vi "Instrument Name and Icon UI.vi"(11 "Template Name":string="Framework-Template") -> ()   [LabVIEW 2019, in "ProjectItem.lvclass"]
uses:
  ProjectItem.lvclass
  Typedefs/ClassData--Cluster.ctl
  <vilib>/LabVIEW Icon API/lv_icon/Classes/Icon/Icon.lvclass
  <vilib>/LabVIEW Icon API/LabVIEW Icon API.lvlib
panel:
  in  "Launch Icon Editor":bool
  in  "Cancel":bool
  out "Instrument UI Library Icon":picture
  out "Instrument Library Icon":picture
  in  "OK":bool
  in  "Icon Text":string="NEW"
  in  "New Name":string="NewInstrument"
  in  "Instrument UI Color":u32(colorbox)=12123647
  in  "Instrument UI Text Color":u32(colorbox)
  in  "Instrument Color":u32(colorbox)=6618880
  in  "Instrument Text Color":u32(colorbox)
  # "1. Rename your new project and classes"
  # "2. Design a new icon"
  # "3. Write out"
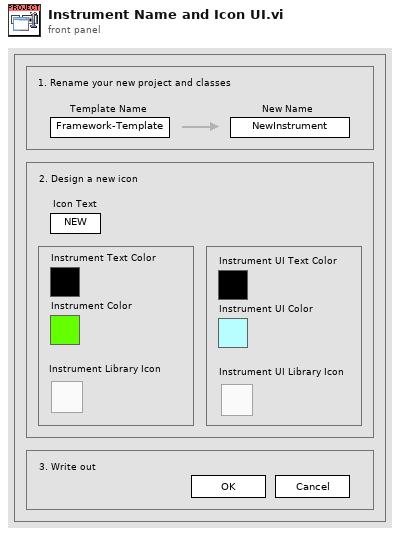
[diagram p1: front panel]
types:
  T1 = enum32{"Invalid", "Standard", "Closed", "Hidden", "Minimized", "Maximized"}
  T2 = enum32{"invalid app kind", "Development System", "Run Time System", "Student Edition", "Embedded LabVIEW", "Evaluation", "Custom"}
  T3 = typedef "ProjectItem.lvclass/ClassData--Cluster.ctl" = cluster{"Name":string, "Icon Text":string, "Text Color":u32, "Color":u32, "Icon":refnum<class "Icon.lvclass">}
  T4 = cluster{"Core":cluster{"Current VI Reference":refnum<vi>, "Close Panel on Exit?":bool}, "Replace Template":string, "Instrument":T3, "Instrument UI":T3, "ProjectItem":refnum<class "ProjectItem.lvclass">}
  T5 = cluster{"Current VI Reference":refnum<vi>, "Close Panel on Exit?":bool}
  T6 = typedef "imagedata.ctl" = cluster{"image type":i32, "image depth":i32, "image":u8[], "mask":u8[], "colors":u32[], "Rectangle":cluster{"left":i16, "top":i16, "right":i16, "bottom":i16}}
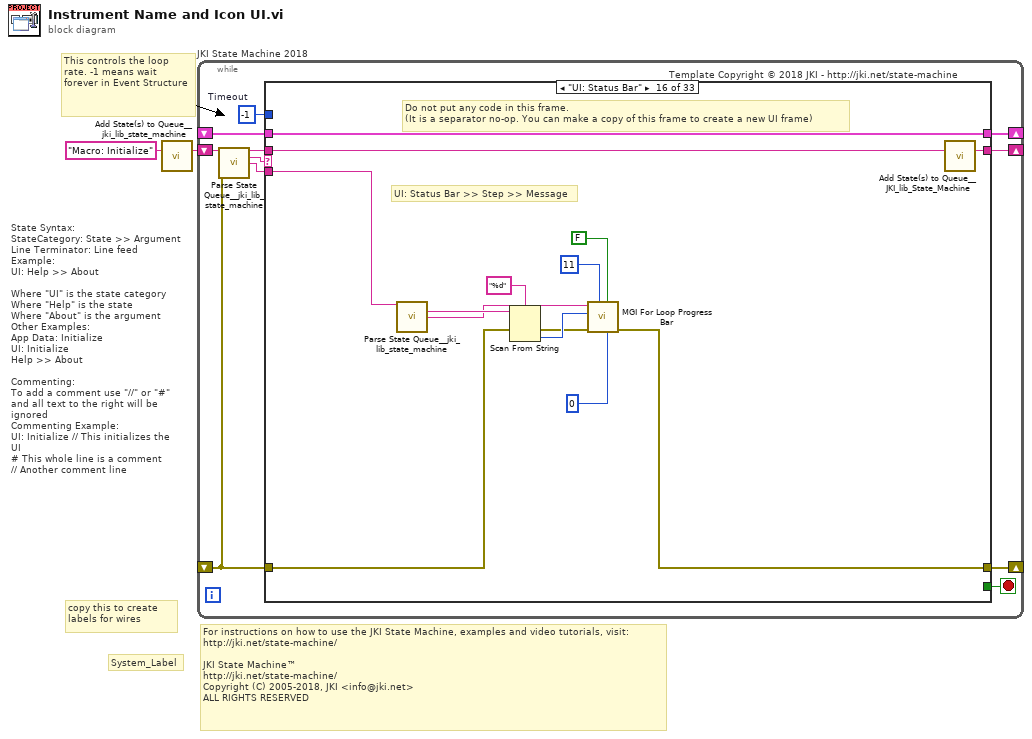
[diagram p0: block diagram]
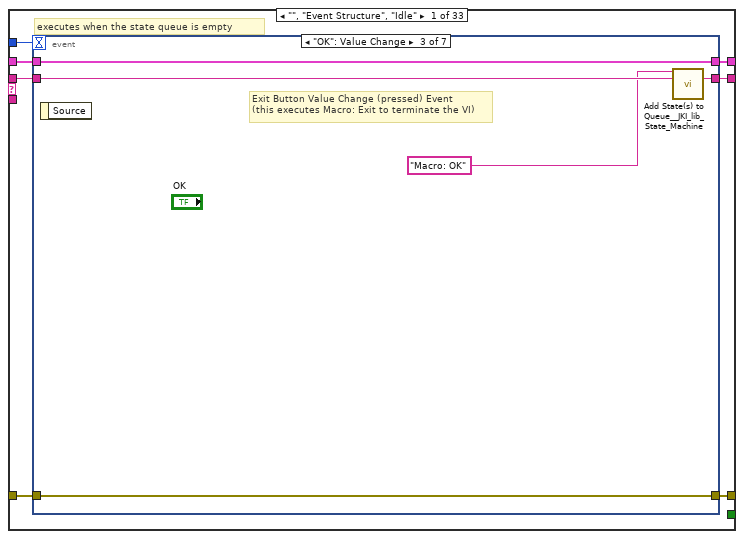
[diagram p2: hidden frame]
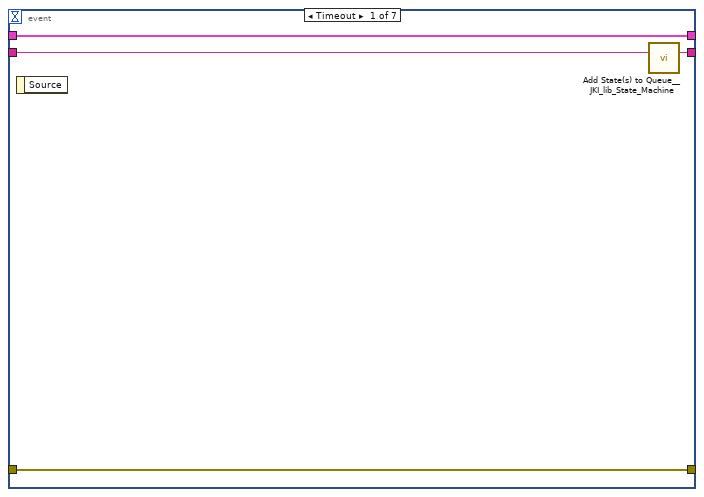
[diagram p3: hidden frame]
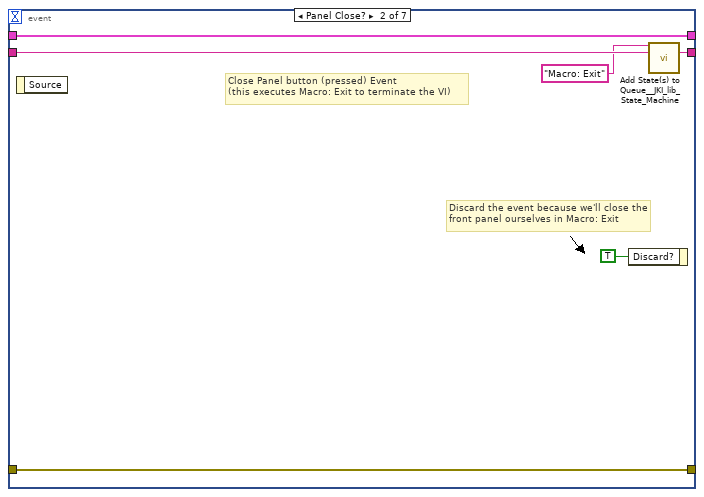
[diagram p4: hidden frame]
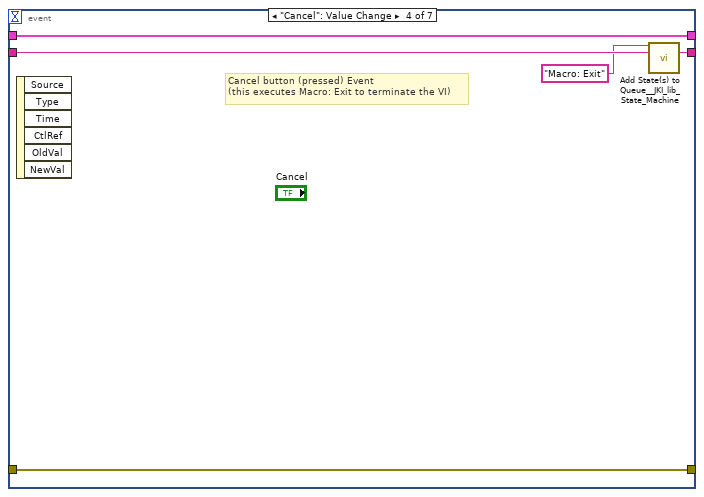
[diagram p5: hidden frame]
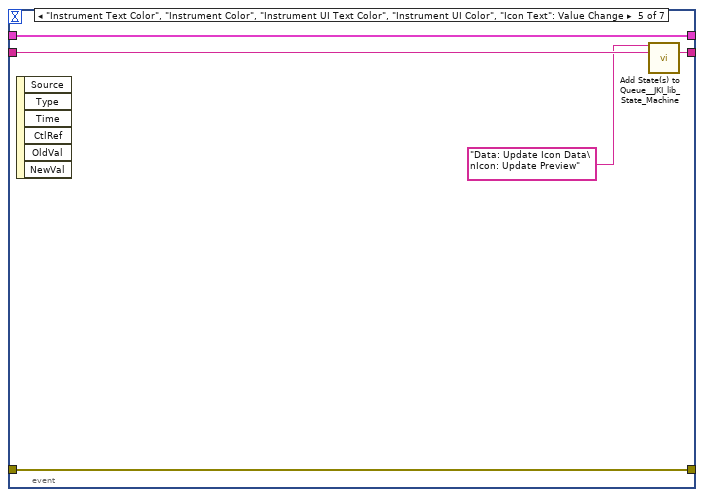
[diagram p6: hidden frame]
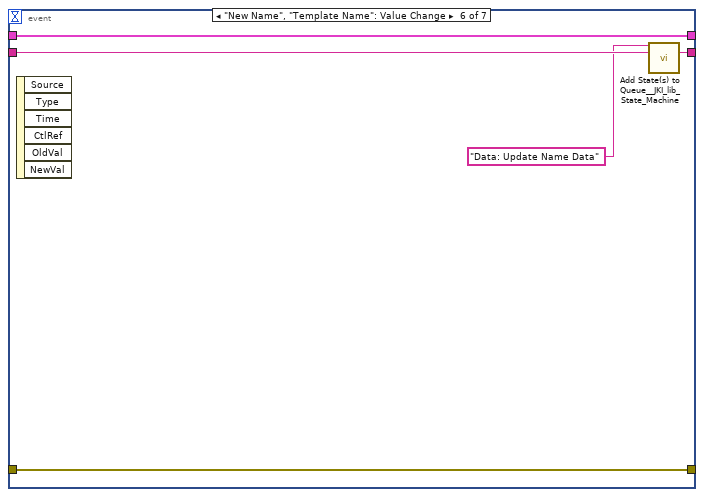
[diagram p7: hidden frame]
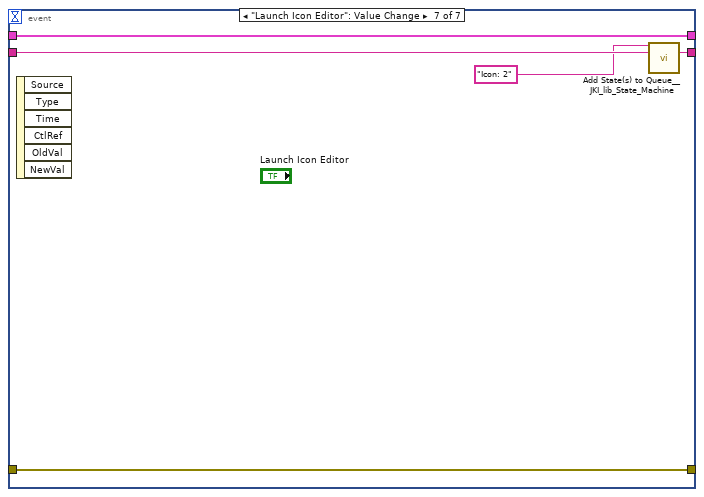
[diagram p8: hidden frame]
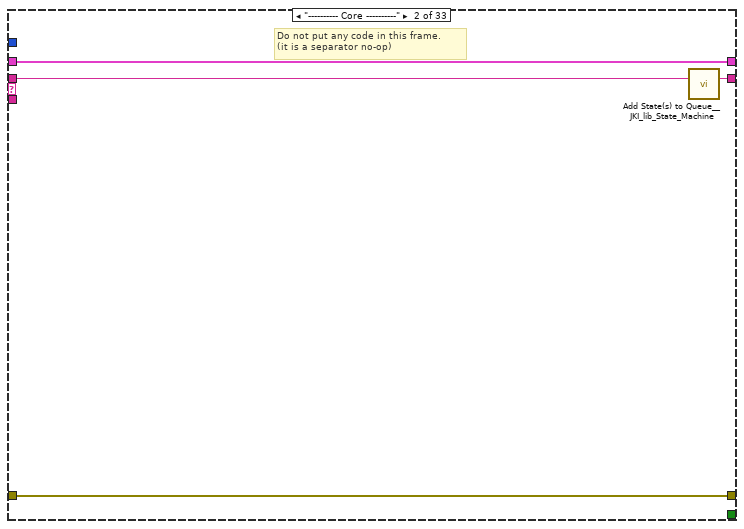
[diagram p9: hidden frame]
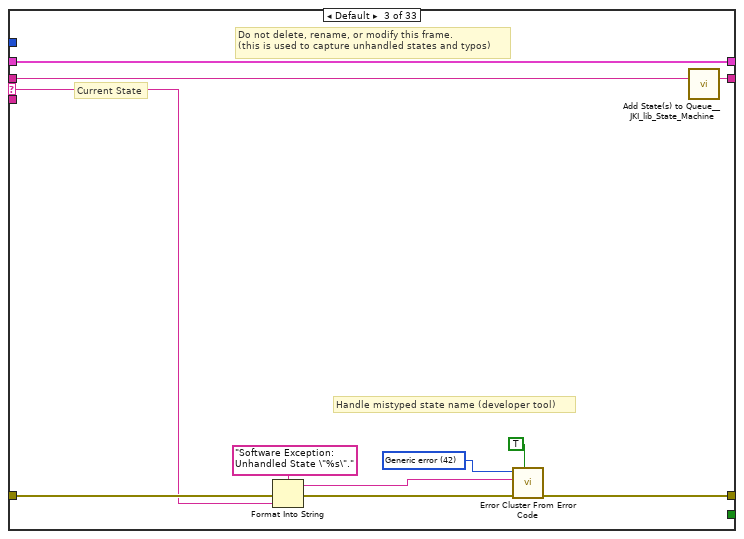
[diagram p10: hidden frame]
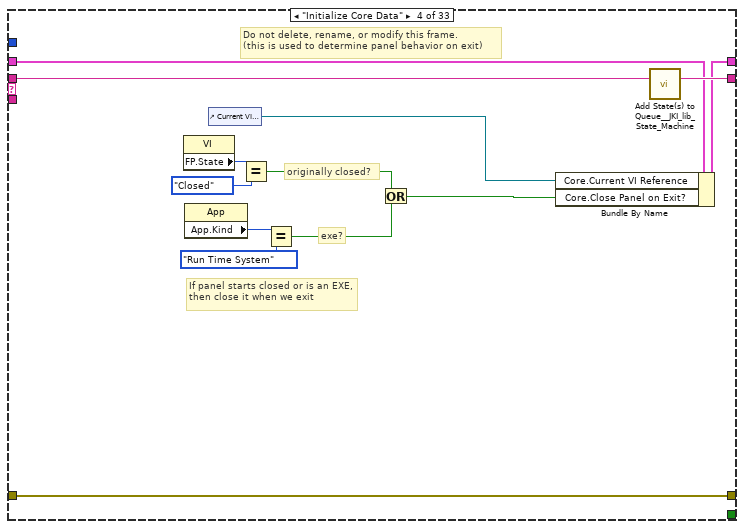
[diagram p11: hidden frame]
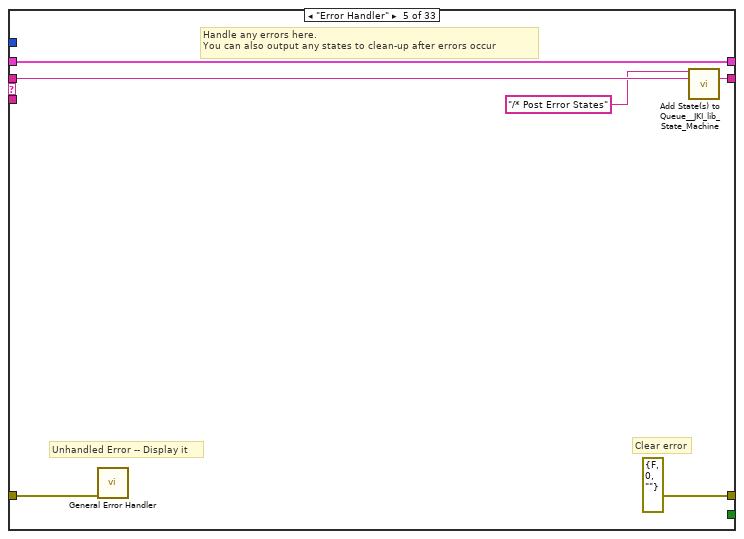
[diagram p12: hidden frame]
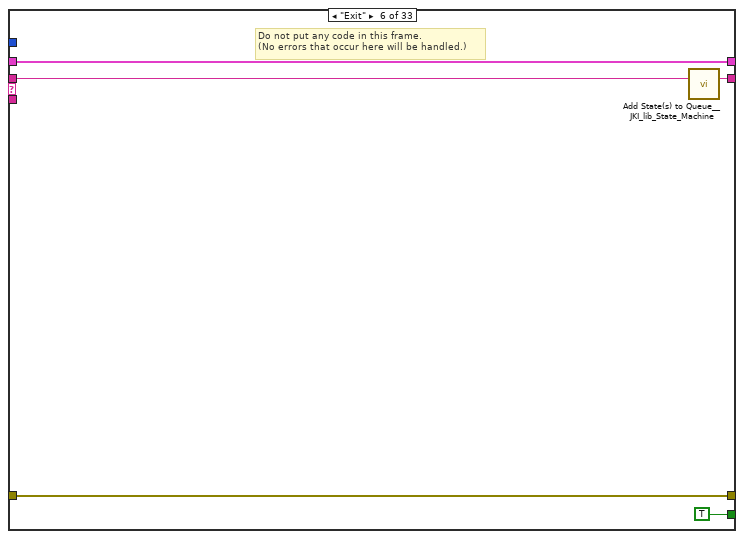
[diagram p13: hidden frame]
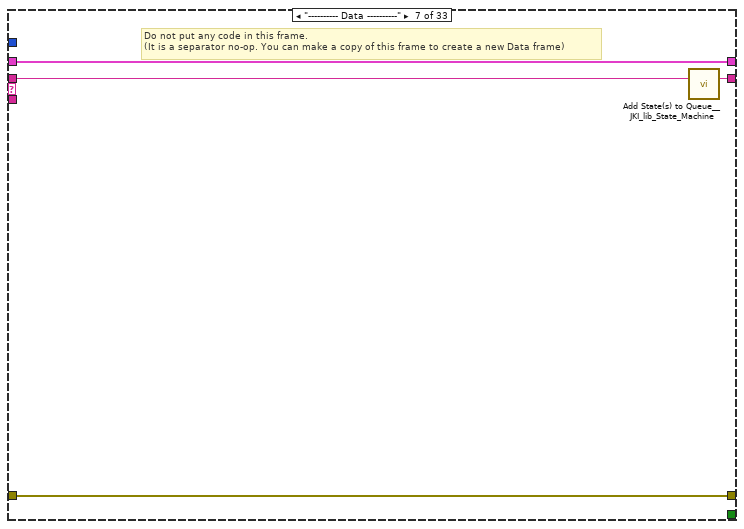
[diagram p14: hidden frame]
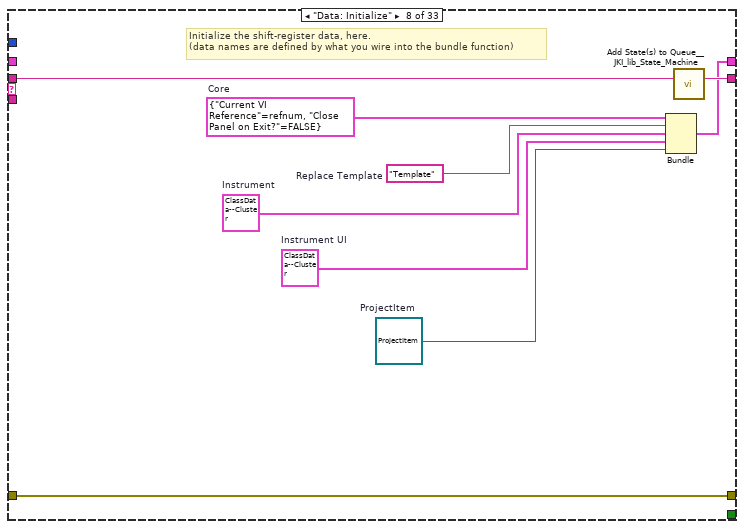
[diagram p15: hidden frame]
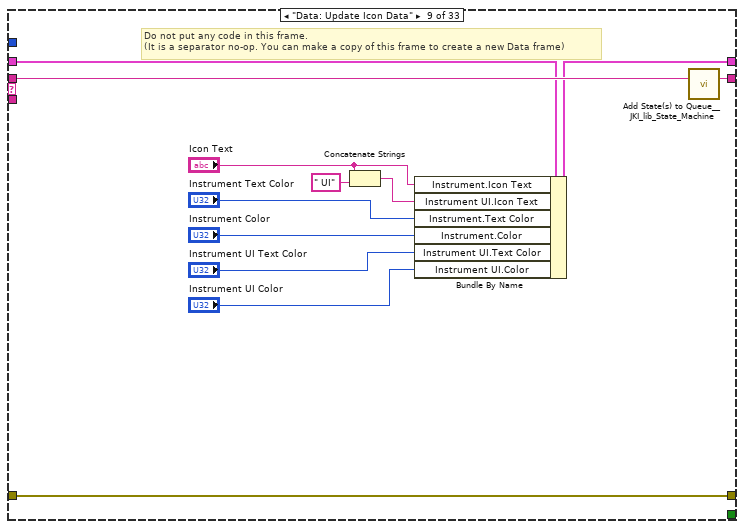
[diagram p16: hidden frame]
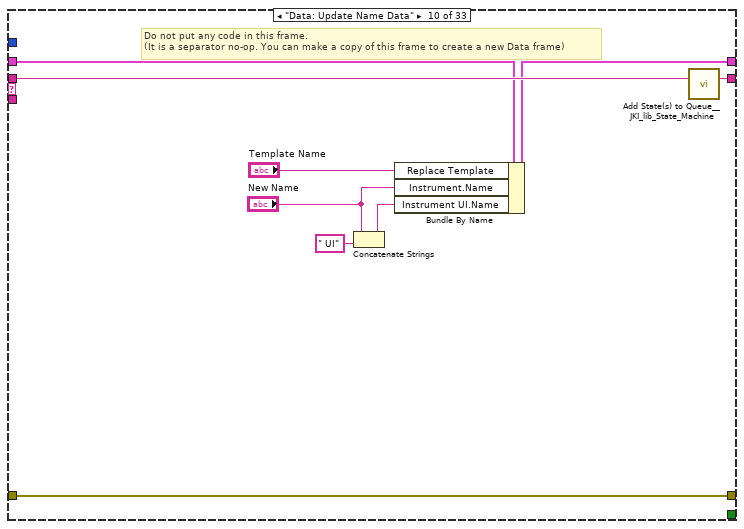
[diagram p17: hidden frame]
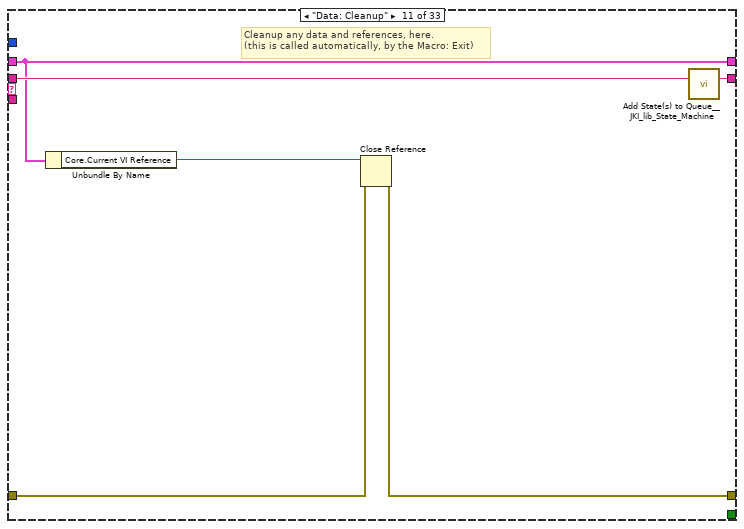
[diagram p18: hidden frame]
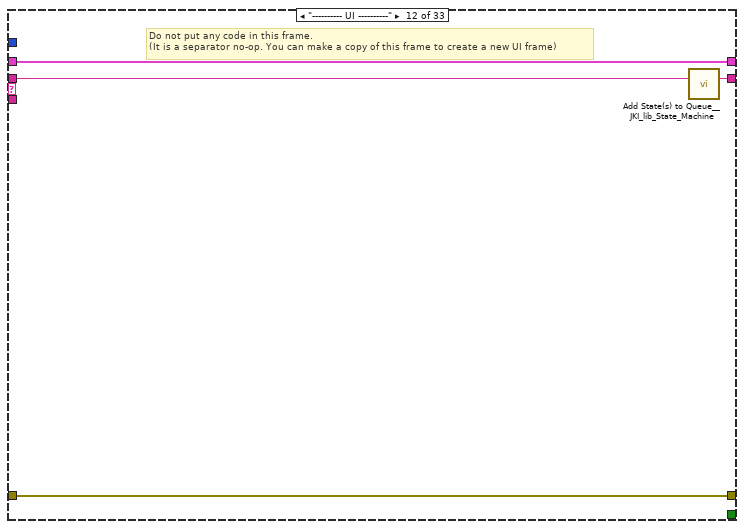
[diagram p19: hidden frame]
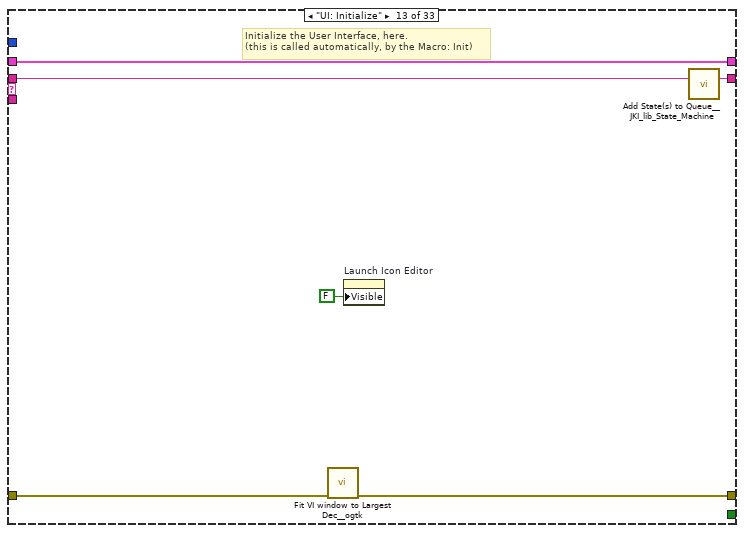
[diagram p20: hidden frame]
diagram:
  # "For instructions on how to use the JKI State Machine, examples and video tutorials, visit:\nhttp://jki.net/state-machine/\n\nJKI State Machine™\nhttp://jki.net/state-machine/\nCopyright (C) 2005-2018, JKI <info@jki.net>\nALL RIGHTS RESERVED"
  # "State Syntax:\nStateCategory: State >> Argument\nLine Terminator: Line feed\nExample:\nUI: Help >> About\n\nWhere \"UI\" is the state category\nWhere \"Help\" is the state\nWhere \"About\" is the argument\nOther Examples:\nApp Data: Initialize\nUI: Initialize\nHelp >> About\n\nCommenting:\nTo add a comment use \"//\" or \"#\" and all text to the right will be ignored\nCommenting Example:\nUI: Initialize // This initializes the UI\n# This whole line is a comment\n// Another comment line"
  # "copy this to create labels for wires"
  # "This controls the loop rate. -1 means wait forever in Event Structure"
  # "System_Label"
  n1 = call <vilib>:"Add State(s) to Queue__jki_lib_state_machine.vi"("State(s) in (\"\")"="Macro: Initialize") -> ("States Out"=w2:string)  [unwired: 14 in]
  n2 = while "JKI State Machine 2018" {
    shift-right: [w6] -> _
    shift-left: _ -> [w5]
    shift-right: [w9] -> _
    shift-left: _ -> [w3]
    shift-right: [w8] -> _
    shift-left: w2 -> [w10]
    stop <- w7 stop-if-true
    w4 = -1  # Timeout
    # "Template Copyright © 2018 JKI - http://jki.net/state-machine"
    n3 = call <vilib>:"Parse State Queue__jki_lib_state_machine.vi"("State Queue"=w10, "Error In (no error)"=w3) -> ("Remaining States"=w12:string, "Current State"=w13:string, "Arguments"=w11:string)  [unwired: 11 in]
    n4 = case shown="\"UI: Status Bar\"" w13 {
      selector: w13 -> [_ _ w60 _ _ _ _ _ _ _ _ _ _ _ _ _ _ _ _ _ _ _ _ _ _ _ _ _ _ _ _ _ _]
      tunnel: w12 -> [w20 w59 w64 w83 w89 w94 w98 w107 w119 w128 w134 w138 w144 w150 w161 w240 w244 w249 w265 w281 w285 w305 w320 w324 w334 w342 w350 w358 w366 w374 w384 w394 w400]
      tunnel: w11 -> [_ _ _ _ _ _ _ _ _ _ _ _ _ w145 w155 w237 _ _ _ _ _ _ _ _ _ _ _ _ _ _ _ _ _]
      tunnel: w5 -> [w18 w56 w62 w76 w86 w92 w95 _ w114 w125 w130 w135 w142 w148 w157 w238 w241 w246 w262 w278 w282 w296 w310 w321 w330 w339 w347 w355 w363 w371 w379 w389 w398]
      tunnel: [w17 w57 w66 w80 errorcluster {"status"=FALSE, "code"=0, "source"=""} ("error out") w91 w96 w104 w117 w126 w131 w136 w141 w146 w158 w228 w242 w247 w263 w279 w283 w299 w312 w322 w327 w336 w344 w351 w359 w367 w381 w391 w395] -> w9
      tunnel: w3 -> [w16 w57 w65 w80 w85 w91 w96 w104 w117 w126 w129 w136 w140 w147 w159 w229 w242 w247 w263 w279 w283 w301 w317 w322 w326 w335 w343 w352 w360 w368 w382 w392 w396]
      tunnel: [w19 w58 w63 w82 w88 w93 w97 w106 w118 w127 w133 w137 w143 w149 w160 w239 w243 w248 w264 w280 w284 w304 w319 w323 w333 w341 w349 w357 w365 w373 w383 w393 w399] -> w8
      tunnel: [_ _ _ _ _ TRUE _ _ _ _ _ _ _ _ _ _ _ _ _ _ _ _ _ _ _ _ _ _ _ _ _ _ _] -> w7
      tunnel: [w15 w56 w62 w81 w86 w92 w95 w105 w113 w124 w130 w135 w142 w148 w157 w238 w241 w246 w262 w278 w282 w297 w316 w321 w329 w338 w346 w354 w362 w370 w380 w390 w398] -> w6
      tunnel: w4 -> [w14 _ _ _ _ _ _ _ _ _ _ _ _ _ _ _ _ _ _ _ _ _ _ _ _ _ _ _ _ _ _ _ _]
      frame "", "Event Structure", "Idle" {
        # "executes when the state queue is empty"
        n5 = event shown="[2] \"OK\": Value Change" {
          selector: _ -> [_ _ _ _ _ _ _]
          dyn-events: _ -> [_ _ _ _ _ _ _]
          timeout: w14 -> [_ _ _ _ _ _ _]
          tunnel: w20 -> [w24 w30 w35 w40 w45 w50 w55]
          tunnel: [w23 w29 w34 w39 w44 w49 w54] -> w19
          tunnel: w18 -> [w21 w27 w32 w37 w41 w46 w51]
          tunnel: [w22 w28 w33 w38 w43 w48 w53] -> w17
          tunnel: w16 -> [w22 w28 w33 w38 w43 w48 w53]
          tunnel: [w21 w27 w32 w37 w41 w46 w51] -> w15
          event Timeout {
            n6 = event-data() -> ()  [unwired: 1 in, 1 out]
            n7 = call <vilib>:"Add State(s) to Queue__JKI_lib_State_Machine.vi"("State(s) in (\"\")"=w24) -> ("States Out"=w23:string)  [unwired: 14 in]
          }
          event Panel Close? {
            # "Discard the event because we'll close the front panel ourselves in Macro: Exit"
            # "Close Panel button (pressed) Event\n(this executes Macro: Exit to terminate the VI)"
            n8 = event-data() -> ()  [unwired: 1 in, 1 out]
            n9 = event-data("Discard?"=TRUE) -> ()  [unwired: 1 in, 1 out]
            n10 = call <vilib>:"Add State(s) to Queue__JKI_lib_State_Machine.vi"("State(s) in Front (\"\")"="Macro: Exit", "State(s) in (\"\")"=w30) -> ("States Out"=w29:string)  [unwired: 13 in]
          }
          event "OK": Value Change {
            # "Exit Button Value Change (pressed) Event\n(this executes Macro: Exit to terminate the VI)"
            n11 = event-data() -> ()  [unwired: 1 in, 1 out]
            n12 = call <vilib>:"Add State(s) to Queue__JKI_lib_State_Machine.vi"("State(s) in Front (\"\")"="Macro: OK", "State(s) in (\"\")"=w35) -> ("States Out"=w34:string)  [unwired: 13 in]
          }
          event "Cancel": Value Change {
            # "Cancel button (pressed) Event\n(this executes Macro: Exit to terminate the VI)"
            n13 = event-data() -> ()  [unwired: 1 in, 6 out]
            n14 = call <vilib>:"Add State(s) to Queue__JKI_lib_State_Machine.vi"("State(s) in Front (\"\")"="Macro: Exit", "State(s) in (\"\")"=w40) -> ("States Out"=w39:string)  [unwired: 13 in]
          }
          event "Instrument Text Color", "Instrument Color", "Instrument UI Text Color", "Instrument UI Color", "Icon Text": Value Change {
            n15 = event-data() -> ()  [unwired: 1 in, 6 out]
            n16 = call <vilib>:"Add State(s) to Queue__JKI_lib_State_Machine.vi"("State(s) in Front (\"\")"="Data: Update Icon Data\nIcon: Update Preview", "State(s) in (\"\")"=w45) -> ("States Out"=w44:string)  [unwired: 13 in]
          }
          event "New Name", "Template Name": Value Change {
            n17 = event-data() -> ()  [unwired: 1 in, 6 out]
            n18 = call <vilib>:"Add State(s) to Queue__JKI_lib_State_Machine.vi"("State(s) in Front (\"\")"="Data: Update Name Data", "State(s) in (\"\")"=w50) -> ("States Out"=w49:string)  [unwired: 13 in]
          }
          event "Launch Icon Editor": Value Change {
            n19 = event-data() -> ()  [unwired: 1 in, 6 out]
            n20 = call <vilib>:"Add State(s) to Queue__JKI_lib_State_Machine.vi"("State(s) in Front (\"\")"="Icon: 2", "State(s) in (\"\")"=w55) -> ("States Out"=w54:string)  [unwired: 13 in]
          }
        }
      }
      frame "---------- Core ----------" {
        # "Do not put any code in this frame.\n(it is a separator no-op)"
        n21 = call <vilib>:"Add State(s) to Queue__JKI_lib_State_Machine.vi"("State(s) in (\"\")"=w59) -> ("States Out"=w58:string)  [unwired: 14 in]
      }
      frame Default {
        w69 = 42 items=["No error", "Argument error", "Memory is full", "Out of zone", "End of file", "File already open", "Generic file I/O error", "File not found", "File permission error", "Disk is full", "Duplicate path", "Too many files open", "System feature not enabled", "Resource file not found", "Cannot add resource", "Resource not found", "Image not found", "Image memory error", "Pen does not exist", "Config type invalid", "Config token not found", "Config parse error", "Config memory error", "Bad external code format", "Bad external code offset", "External code not present", "Null window", "Destroy window error", "Null menu", "Print aborted", "Bad print record", "Print driver error", "Windows error during printing", "Memory error during printing", "Print dialog error", "Generic print error", "Invalid device refnum", "Device not found", "Device parameter error", "Device unit error", "Cannot open device", "Device call aborted", "Generic error", "Cancelled by user", "Object ID too low", "Object ID too high", "Object not in heap", "Unknown heap", "Unknown object (invalid DefProc)", "Unknown object (DefProc not in table)", "Message out of range", "Invalid (null) method", "Unknown message", "Manager call not supported", "Bad address", "Network operation in progress", "Network operation timed out", "Connection is busy", "Network attribute not supported", "Network error", "Address in use", "System out of memory", "Connection aborted", "Connection refused", "Not connected", "Already connected", "Connection closed", "Initialization error (interapplication manager)", "Bad occurrence", "Wait on unbound occurrence handler", "Occurrence queue overflow", "Datalog type conflict", "Unused", "Unrecognized type (interapplication manager)", "Memory corrupt", "Failed to make temporary DLL", "Old CIN version", "Drag socket not found", "Failed to load drop-object", "Failed to register OLE object", "Failed to release OLE object", "Format specifier type mismatch", "Unknown format specifier", "Too few format specifiers", "Too many format specifiers", "Scan failed", "Newer CIN version", "Error converting to variant", "Runtime menu error", "Password tampered", "Variant attribute not found", "Incompatible variant data type", "Event data is not available", "Event Store is not present", "Occurrence is not found", "Event Queue is not created", "Event info is not available", "Refnum passed is NULL", "Error retrieving Class GUID", "Error retrieving CoClass GUID", "Error retrieving TypeLib GUID.", "Bad built application magic bytes.", "Specific driver is different from the specific driver associated with the Logical Name.", "There is no session opened to the class driver.", "Max Error", "MAX - Error with config objects", "MAX - Error loading configuration", "MAX - Group not supported"]
        # "Current State"
        # "Do not delete, rename, or modify this frame.\n(this is used to capture unhandled states and typos)"
        # "Handle mistyped state name (developer tool)"
        n22 = Format Into String(format string="Software Exception: Unhandled State \"%s\"." ("message"), error in=w65, w60) -> (resulting string=w68:string, error out=w67:errorcluster)  [unwired: 1 in]
        n23 = call <vilib>:"Error Cluster From Error Code.vi"("show call chain? (False)"=TRUE, "error in (no error)"=w67, "error message (\"\")"=w68, "error code (0)"=w69) -> ("error out"=w66:errorcluster)  [unwired: 5 in]
        n24 = call <vilib>:"Add State(s) to Queue__JKI_lib_State_Machine.vi"("State(s) in (\"\")"=w64) -> ("States Out"=w63:string)  [unwired: 14 in]
      }
      frame "Initialize Core Data" {
        # "Do not delete, rename, or modify this frame.\n(this is used to determine panel behavior on exit)"
        # "originally closed?"
        # "exe?"
        # "If panel starts closed or is an EXE, then close it when we exit"
        n25 = property class="VI"() -> ("FP.State"=w73:T1)  [unwired: 2 in, 2 out]
        n26 = property class="App"() -> ("App.Kind"=w79:T2)  [unwired: 2 in, 2 out]
        n27 = control-ref of="Current VI Reference"() -> (w74:refnum<vi>)
        n28 = Equal?(x=w73, y=T1."Closed" ("Front Panel Window:State")) -> (x = y?=w71:bool)
        n29 = Equal?(x=w79, y=T2."Run Time System" ("Application:Kind")) -> (x = y?=w77:bool)
        n30 = Or(x=w71, y=w77) -> (x .or. y?=w75:bool)
        n31 = Bundle By Name(cluster=w76, "Core.Current VI Reference"=w74, "Core.Close Panel on Exit?"=w75) -> (w81:T4)
        n32 = call <vilib>:"Add State(s) to Queue__JKI_lib_State_Machine.vi"("State(s) in (\"\")"=w83) -> ("States Out"=w82:string)  [unwired: 14 in]
      }
      frame "Error Handler" {
        # "Unhandled Error -- Display it"
        # "Handle any errors here.\nYou can also output any states to clean-up after errors occur"
        # "Clear error"
        n33 = call <vilib>:"General Error Handler.vi"("error in (no error)"=w85) -> ()  [unwired: 10 in, 5 out]
        n34 = call <vilib>:"Add State(s) to Queue__JKI_lib_State_Machine.vi"("State(s) in Front (\"\")"="/* Post Error States", "State(s) in (\"\")"=w89) -> ("States Out"=w88:string)  [unwired: 13 in]
      }
      frame "Exit" {
        # "Do not put any code in this frame.\n(No errors that occur here will be handled.)"
        n35 = call <vilib>:"Add State(s) to Queue__JKI_lib_State_Machine.vi"("State(s) in (\"\")"=w94) -> ("States Out"=w93:string)  [unwired: 14 in]
      }
      frame "---------- Data ----------" {
        # "Do not put any code in this frame.\n(It is a separator no-op. You can make a copy of this frame to create a new Data frame)"
        n36 = call <vilib>:"Add State(s) to Queue__JKI_lib_State_Machine.vi"("State(s) in (\"\")"=w98) -> ("States Out"=w97:string)  [unwired: 14 in]
      }
      frame "Data: Initialize" {
        w99 = T3 {"Name"="NewInstrument", "Icon Text"="NewInstrument", "Text Color"=6618880, "Color"=6618880, "Icon"=refnum}  # Instrument UI
        w101 = refnum<class "ProjectItem.lvclass"> refnum  # ProjectItem
        w102 = T3 {"Name"="NewInstrument", "Icon Text"="NewInstrument", "Text Color"=6618880, "Color"=6618880, "Icon"=refnum}  # Instrument
        w100 = "Template"  # Replace Template
        w103 = T5 {"Current VI Reference"=refnum, "Close Panel on Exit?"=FALSE}  # Core
        # "Initialize the shift-register data, here.\n(data names are defined by what you wire into the bundle function)"
        n37 = Bundle("Core"=w103, "Replace Template"=w100, "Instrument"=w102, "Instrument UI"=w99, "ProjectItem"=w101) -> (w105:T4)  [unwired: 1 in]
        n38 = call <vilib>:"Add State(s) to Queue__JKI_lib_State_Machine.vi"("State(s) in (\"\")"=w107) -> ("States Out"=w106:string)  [unwired: 14 in]
      }
      frame "Data: Update Icon Data" {
        # "Do not put any code in this frame.\n(It is a separator no-op. You can make a copy of this frame to create a new Data frame)"
        n39 = Concatenate Strings("Icon Text", " UI" ("string")) -> (w108:string)
        n40 = Bundle By Name(cluster=w114, "Instrument.Icon Text"="Icon Text", "Instrument UI.Icon Text"=w108, "Instrument.Text Color"="Instrument Text Color", "Instrument.Color"="Instrument Color", "Instrument UI.Text Color"="Instrument UI Text Color", "Instrument UI.Color"="Instrument UI Color") -> (w113:T4)
        n41 = call <vilib>:"Add State(s) to Queue__JKI_lib_State_Machine.vi"("State(s) in (\"\")"=w119) -> ("States Out"=w118:string)  [unwired: 14 in]
      }
      frame "Data: Update Name Data" {
        # "Do not put any code in this frame.\n(It is a separator no-op. You can make a copy of this frame to create a new Data frame)"
        n42 = Concatenate Strings("New Name", " UI" ("string")) -> (w121:string)
        n43 = Bundle By Name(cluster=w125, "Replace Template"="Template Name", "Instrument.Name"="New Name", "Instrument UI.Name"=w121) -> (w124:T4)
        n44 = call <vilib>:"Add State(s) to Queue__JKI_lib_State_Machine.vi"("State(s) in (\"\")"=w128) -> ("States Out"=w127:string)  [unwired: 14 in]
      }
      frame "Data: Cleanup" {
        # "Cleanup any data and references, here.\n(this is called automatically, by the Macro: Exit)"
        n45 = Unbundle By Name(w130) -> ("Core.Current VI Reference"=w132:refnum<vi>)
        n46 = Close Reference(reference=w132, error in (no error)=w129) -> (error out=w131:errorcluster)
        n47 = call <vilib>:"Add State(s) to Queue__JKI_lib_State_Machine.vi"("State(s) in (\"\")"=w134) -> ("States Out"=w133:string)  [unwired: 14 in]
      }
      frame "---------- UI ----------" {
        # "Do not put any code in this frame.\n(It is a separator no-op. You can make a copy of this frame to create a new UI frame)"
        n48 = call <vilib>:"Add State(s) to Queue__JKI_lib_State_Machine.vi"("State(s) in (\"\")"=w138) -> ("States Out"=w137:string)  [unwired: 14 in]
      }
      frame "UI: Initialize" {
        # "Initialize the User Interface, here.\n(this is called automatically, by the Macro: Init)"
        n49 = call <userlib>:"Fit VI window to Largest Dec__ogtk.vi"("error in (no error)"=w140) -> ("error out"=w141:errorcluster)  [unwired: 5 in, 1 out]
        n50 = property on="Launch Icon Editor" class="Bool"("Visible"=FALSE) -> ()  [unwired: 2 in, 2 out]
        n51 = call <vilib>:"Add State(s) to Queue__JKI_lib_State_Machine.vi"("State(s) in (\"\")"=w144) -> ("States Out"=w143:string)  [unwired: 14 in]
      }
      frame "UI: Cursor Set" {
        # "Argument"
        # "Set and Unset Cursor Busy.\n(Usage: \"UI: Cursor Set >> Busy|Idle\")"
        n52 = case shown="\"Idle\", Default" w145 {
          tunnel: w147 -> [w152 w154]
          tunnel: [w151 w153] -> w146
          frame "Idle", Default {
            n53 = call <vilib>:"Unset Busy.vi"("error in (no error)"=w152) -> ("error out"=w151:errorcluster)  [unwired: 10 in]
          }
          frame "Busy" {
            n54 = call <vilib>:"Set Busy.vi"("error in (no error)"=w154) -> ("error out"=w153:errorcluster)  [unwired: 9 in, 1 out]
          }
        }
        n55 = call <vilib>:"Add State(s) to Queue__JKI_lib_State_Machine.vi"("State(s) in (\"\")"=w150) -> ("States Out"=w149:string)  [unwired: 14 in]
      }
      frame "UI: Front Panel State" {
        # "Argument"
        # "Set Front Panel Open or Closed\n(Usage: \"UI: Front Panel State >> Open|Close\")"
        n56 = Unbundle By Name(w157) -> ("Core.Current VI Reference"=w156:refnum<vi>)
        n57 = case shown="\"Minimize\", \"Minimized\"" w155 {
          tunnel: w159 -> [w167 w182 w193 w206 w219]
          tunnel: [w169 w183 w195 w208 w221] -> w158
          tunnel: w156 -> [w168 w180 w194 w207 w220]
          frame "Open", "Standard", Default {
            w162 = T1."Standard" ("State")
            n58 = property class="VI"(reference=w168, error in=w167) -> (reference out=w165:refnum<vi>, error out=w166:errorcluster, "FP.State"=w164:T1)
            n59 = Not Equal?(x=w164, y=w162) -> (x != y?=w163:bool)
            n60 = case shown="True" w163 {
              tunnel: [w173 w175] -> w169
              tunnel: w166 -> [w172 w175]
              tunnel: w165 -> [w171 _]
              tunnel: w162 -> [w170 _]
              frame True {
                n61 = invoke class="VI" method="FP.Open"(reference=w171, error in=w172, "Activate"=TRUE, "State"=w170) -> (error out=w173:errorcluster)  [unwired: 1 in, 4 out]
              }
              frame False {
              }
            }
          }
          frame "Close", "Closed" {
            n62 = property class="VI"(reference=w180, error in=w182) -> (reference out=w179:refnum<vi>, error out=w181:errorcluster, "FP.State"=w177:T1)
            n63 = Not Equal?(x=w177, y=T1."Closed" ("Front Panel Window:State")) -> (x != y?=w176:bool)
            n64 = case shown="True" w176 {
              tunnel: [w184 w187] -> w183
              tunnel: w181 -> [w184 w186]
              tunnel: w179 -> [_ w185]
              frame False {
              }
              frame True {
                n65 = invoke class="VI" method="FP.Close"(reference=w185, error in=w186) -> (error out=w187:errorcluster)  [unwired: 1 in, 2 out]
              }
            }
          }
          frame "Hidden", "Hide" {
            w188 = T1."Hidden" ("State")
            n66 = property class="VI"(reference=w194, error in=w193) -> (reference out=w191:refnum<vi>, error out=w192:errorcluster, "FP.State"=w190:T1)
            n67 = Not Equal?(x=w190, y=w188) -> (x != y?=w189:bool)
            n68 = case shown="True" w189 {
              tunnel: [w199 w200] -> w195
              tunnel: w192 -> [w198 w200]
              tunnel: w191 -> [w197 _]
              tunnel: w188 -> [w196 _]
              frame True {
                n69 = invoke class="VI" method="FP.Open"(reference=w197, error in=w198, "State"=w196) -> (error out=w199:errorcluster)  [unwired: 2 in, 4 out]
              }
              frame False {
              }
            }
          }
          frame "Minimize", "Minimized" {
            w201 = T1."Minimized" ("State")
            n70 = property class="VI"(reference=w207, error in=w206) -> (reference out=w204:refnum<vi>, error out=w205:errorcluster, "FP.State"=w203:T1)
            n71 = Not Equal?(x=w203, y=w201) -> (x != y?=w202:bool)
            n72 = case shown="True" w202 {
              tunnel: [w212 w213] -> w208
              tunnel: w205 -> [w211 w213]
              tunnel: w204 -> [w210 _]
              tunnel: w201 -> [w209 _]
              frame True {
                n73 = invoke class="VI" method="FP.Open"(reference=w210, error in=w211, "State"=w209) -> (error out=w212:errorcluster)  [unwired: 2 in, 4 out]
              }
              frame False {
              }
            }
          }
          frame "Maximize", "Maximized" {
            w214 = T1."Maximized" ("State")
            n74 = property class="VI"(reference=w220, error in=w219) -> (reference out=w217:refnum<vi>, error out=w218:errorcluster, "FP.State"=w216:T1)
            n75 = Not Equal?(x=w216, y=w214) -> (x != y?=w215:bool)
            n76 = case shown="True" w215 {
              tunnel: [w225 w226] -> w221
              tunnel: w218 -> [w224 w226]
              tunnel: w217 -> [w223 _]
              tunnel: w214 -> [w222 _]
              frame True {
                n77 = invoke class="VI" method="FP.Open"(reference=w223, error in=w224, "State"=w222) -> (error out=w225:errorcluster)  [unwired: 2 in, 4 out]
              }
              frame False {
              }
            }
          }
        }
        n78 = call <vilib>:"Add State(s) to Queue__JKI_lib_State_Machine.vi"("State(s) in (\"\")"=w161) -> ("States Out"=w160:string)  [unwired: 14 in]
      }
      frame "UI: Status Bar" {
        # "UI: Status Bar >> Step >> Message"
        # "Do not put any code in this frame.\n(It is a separator no-op. You can make a copy of this frame to create a new UI frame)"
        n79 = call <vilib>:"Parse State Queue__jki_lib_state_machine.vi"("State Queue"=w237) -> ("Current State"=w233:string, "Arguments"=w232:string)  [unwired: 12 in, 1 out]
        n80 = Scan From String(format string="%d", input string=w233, error in=w229) -> (error out=w230:errorcluster, output 1=w236:i32)  [unwired: 2 in, 2 out]
        n81 = call <userlib>:"MGI For Loop Progress Bar.vi"("Wait Time (ms) (1000)"=u32 0, "Show Time? (T)"=FALSE, "Total Iter"=11, "error in (no error)"=w230, "Current Iter"=w236, "Message"=w232) -> ("error out"=w228:errorcluster)  [unwired: 4 in, 1 out]
        n82 = call <vilib>:"Add State(s) to Queue__JKI_lib_State_Machine.vi"("State(s) in (\"\")"=w240) -> ("States Out"=w239:string)  [unwired: 14 in]
      }
      frame "---------- Macro ----------" {
        # "Do not put any code in this frame.\n(It is a separator no-op. You can make a copy of this frame to create a new Macro frame)"
        n83 = call <vilib>:"Add State(s) to Queue__JKI_lib_State_Machine.vi"("State(s) in (\"\")"=w244) -> ("States Out"=w243:string)  [unwired: 14 in]
      }
      frame "Macro: Initialize" {
        # "Initialization Macro\n(This is called once, when the VI starts)"
        n84 = call <vilib>:"Add State(s) to Queue__JKI_lib_State_Machine.vi"("State(s) in Front (\"\")"="Data: Initialize\nInitialize Core Data\nUI: Initialize\nUI: Front Panel State >> Open\nData: Update Icon Data\nIcon: Update Preview", "State(s) in (\"\")"=w249) -> ("States Out"=w248:string)  [unwired: 13 in]
      }
      frame "Macro: OK" {
        w256 = "\n" ("delimiter")
        # "Initialization Macro\n(This is called once, when the VI starts)"
        n85 = call <vilib>:"Delimited String to 1D String Array.vi"("delimiter"=w256, "delimited string"="Updating Data Wire\nUpdating Icon Preview\nInitializing References\nRenaming Project File\nRenaming Classes\nRenaming VIs\nRenaming Typedefs\nRenaming GObjects\nUpdating Library and VI Icons\nUpdating Library Wires\nSaving and Closing References\nFinish") -> ("string array"=w260:string[])  [unwired: 9 in]
        n86 = call <vilib>:"Delimited String to 1D String Array.vi"("delimiter"=w256, "delimited string"="Data: Update Name Data\nIcon: Update Preview\nLibrary: Initialize References\nLibrary: Rename Project\nLibrary: Rename Classes\nLibrary: Rename VIs\nLibrary: Rename Controls\nLibrary: Rename GObjects\nLibrary: Update Library Icons\nLibrary: Update Library Wires\nLibrary: Close References") -> ("string array"=w252:string[])  [unwired: 9 in]
        n87 = for {
          tunnel: "UI: Status Bar" ("State") -> [w269]
          tunnel: w260 -> [w266] mode=indexing
          tunnel: [w268] -> w253 mode=indexing
          i -> [w271]
          n88 = Format Into String(w271) -> (resulting string=w267:string)  [unwired: 3 in, 1 out]
          n89 = call <vilib>:"Build State String with Arguments__JKI_lib_State_Machine.vi"("Arguments (\"\")"=w267, "State"=w269) -> ("State with Arguments"=w270:string)  [unwired: 4 in]
          n90 = call <vilib>:"Build State String with Arguments__JKI_lib_State_Machine.vi"("Arguments (\"\")"=w266, "State"=w270) -> ("State with Arguments"=w268:string)  [unwired: 4 in]
        }
        n91 = Interleave 1D Arrays(w253, w252) -> (w255:string[])
        n92 = call <vilib>:"1D String Array to Delimited String.vi"("delimiter"=w256, "string array"=w255) -> ("delimited string"=w254:string)  [unwired: 9 in]
        n93 = call <vilib>:"Add State(s) to Queue__jki_lib_state_machine.vi"("State(s) in Front (\"\")"="UI: Cursor Set >> Busy", "State(s) in (\"\")"=w254, "State(s) at Back (\"\")"="UI: Cursor Set >> Idle\nMacro: Exit") -> ("States Out"=w251:string)  [unwired: 12 in]
        n94 = call <vilib>:"Add State(s) to Queue__JKI_lib_State_Machine.vi"("State(s) in Front (\"\")"=w251, "State(s) in (\"\")"=w265) -> ("States Out"=w264:string)  [unwired: 13 in]
      }
      frame "Macro: Exit" {
        # "Exit Macro\n(This is called once, when the VI exits)"
        n95 = Unbundle By Name(w278) -> ("Core.Close Panel on Exit?"=w277:bool)
        n96 = Select(t="UI: Front Panel State >> Close", s=w277, f="") -> (s? t:f=w274:string)
        n97 = call <vilib>:"Add State(s) to Queue__JKI_lib_State_Machine.vi"("State(s) in (\"\")"=w274, "State(s) at Back (\"\")"="Data: Cleanup\nExit") -> ("States Out"=w272:string)  [unwired: 13 in]
        n98 = call <vilib>:"Add State(s) to Queue__JKI_lib_State_Machine.vi"("State(s) in Front (\"\")"=w272, "State(s) in (\"\")"=w281) -> ("States Out"=w280:string)  [unwired: 13 in]
      }
      frame "---------- Icon ----------" {
        # "Template Separator\n(You can make a copy of, or modify, this frame)"
        n99 = call <vilib>:"Add State(s) to Queue__JKI_lib_State_Machine.vi"("State(s) in (\"\")"=w285) -> ("States Out"=w284:string)  [unwired: 14 in]
      }
      frame "Icon: Update Preview" {
        # "Your code here.\n(You can make a copy of, or modify, this frame)"
        n100 = Unbundle By Name(w296) -> ("Instrument.Icon Text"=w293:string, "Instrument.Icon"=w292:refnum<class "Icon.lvclass">, "Instrument.Text Color"=w303:u32, "Instrument.Color"=w302:u32, "Instrument UI.Icon Text"=w294:string, "Instrument UI.Icon"=w291:refnum<class "Icon.lvclass">, "Instrument UI.Text Color"=w290:u32, "Instrument UI.Color"=w289:u32)
        n101 = case shown="False" FALSE {
          frame False {
          }
          frame True {
            n102 = call <vilib>:"Set Library Icon.vi"("Icon"=refnum<class "Icon.lvclass"> refnum, "Library Refnum in"=refnum<vi> refnum) -> ("error out"=w308:errorcluster, "Library Refnum out"=w309:refnum<vi>)  [unwired: 8 in]
            n103 = call <vilib>:"Get Library Icon.vi"("error in (no error)"=w308, "Library Refnum in"=w309) -> ()  [unwired: 7 in, 3 out]
          }
        }
        n104 = call "Update Icon Preview.vi"("Icon Text"=w293, "error in (no error)"=w301, "Instrument  Color"=w302, "Instrument Text Color"=w303, "Icon.lvclass in"=w292) -> ("error out"=w300:errorcluster, "new picture"=→"Instrument Library Icon":picture, "lv_icon.lvlib:Icon.lvclass out"=w295:refnum<class "Icon.lvclass">)  [unwired: 4 in]
        n105 = call "Update Icon Preview.vi"("Icon Text"=w294, "error in (no error)"=w300, "Instrument  Color"=w289, "Instrument Text Color"=w290, "Icon.lvclass in"=w291) -> ("error out"=w299:errorcluster, "new picture"=→"Instrument UI Library Icon":picture, "lv_icon.lvlib:Icon.lvclass out"=w287:refnum<class "Icon.lvclass">)  [unwired: 4 in]
        n106 = Bundle By Name(cluster=w296, "Instrument.Icon"=w295, "Instrument UI.Icon"=w287) -> (w297:T4)
        n107 = call <vilib>:"Add State(s) to Queue__JKI_lib_State_Machine.vi"("State(s) in (\"\")"=w305) -> ("States Out"=w304:string)  [unwired: 14 in]
      }
      frame "Icon: 2" {
        # "Your code here.\n(You can make a copy of, or modify, this frame)"
        n108 = Unbundle By Name(w310) -> ("Instrument.Icon"=w318:refnum<class "Icon.lvclass">)
        n109 = call <vilib>:"Launch Icon Editor.vi"("error in (no error)"=w317, "Icon in"=w318) -> ("error out"=w313:errorcluster, "Icon out"=w314:refnum<class "Icon.lvclass">)  [unwired: 7 in, 1 out]
        n110 = call <vilib>:"Get Flattened Image.vi"("error in (no error)"=w313, "lv_icon.lvlib:Icon.lvclass in"=w314) -> ("error out"=w312:errorcluster, "Color Image"=w315:T6)  [unwired: 6 in, 2 out]
        n111 = Bundle By Name(cluster=w310, "Instrument.Icon"=w314) -> (w316:T4)
        n112 = call <vilib>:"Draw Flattened Pixmap.vi"("image data"=w315) -> ("new picture"=w311:picture)  [unwired: 8 in]
        n113 = local write "Instrument Library Icon"(w311) -> ()
        n114 = call <vilib>:"Add State(s) to Queue__JKI_lib_State_Machine.vi"("State(s) in (\"\")"=w320) -> ("States Out"=w319:string)  [unwired: 14 in]
      }
      frame "---------- Library ----------" {
        # "Template Separator\n(You can make a copy of, or modify, this frame)"
        n115 = call <vilib>:"Add State(s) to Queue__JKI_lib_State_Machine.vi"("State(s) in (\"\")"=w324) -> ("States Out"=w323:string)  [unwired: 14 in]
      }
      frame "Library: Initialize References" {
        # "Template Separator\n(You can make a copy of, or modify, this frame)"
        n116 = Unbundle By Name(w330) -> ("ProjectItem"=w325:refnum<class "ProjectItem.lvclass">, "Replace Template"=w332:string, "Instrument.Name"=w331:string)
        n117 = call "Initialize.vi"("ProjectItem"=w325, "error in (no error)"=w326, "New Name"=w331, "Pattern"=w332) -> ("error out"=w327:errorcluster, "ProjectItem out"=w328:refnum<class "ProjectItem.lvclass">)  [unwired: 6 in]
        n118 = Bundle By Name(cluster=w330, "ProjectItem"=w328) -> (w329:T4)
        n119 = call <vilib>:"Add State(s) to Queue__JKI_lib_State_Machine.vi"("State(s) in (\"\")"=w334) -> ("States Out"=w333:string)  [unwired: 14 in]
      }
      frame "Library: Rename Project" {
        # "Template Separator\n(You can make a copy of, or modify, this frame)"
        n120 = Unbundle By Name(w339) -> ("ProjectItem"=w340:refnum<class "ProjectItem.lvclass">)  [unwired: 2 out]
        n121 = call "Rename Project.vi"("error in (no error)"=w335, "ProjectItem in"=w340) -> ("error out"=w336:errorcluster, "ProjectItem out"=w337:refnum<class "ProjectItem.lvclass">)  [unwired: 8 in]
        n122 = Bundle By Name(cluster=w339, "ProjectItem"=w337) -> (w338:T4)
        n123 = call <vilib>:"Add State(s) to Queue__JKI_lib_State_Machine.vi"("State(s) in (\"\")"=w342) -> ("States Out"=w341:string)  [unwired: 14 in]
      }
      frame "Library: Rename Classes" {
        # "Template Separator\n(You can make a copy of, or modify, this frame)"
        n124 = Unbundle By Name(w347) -> ("ProjectItem"=w348:refnum<class "ProjectItem.lvclass">)  [unwired: 2 out]
        n125 = call "Rename Classes.vi"("error in (no error)"=w343, "ProjectItem in"=w348) -> ("error out"=w344:errorcluster, "ProjectItem out"=w345:refnum<class "ProjectItem.lvclass">)  [unwired: 8 in]
        n126 = Bundle By Name(cluster=w347, "ProjectItem"=w345) -> (w346:T4)
        n127 = call <vilib>:"Add State(s) to Queue__JKI_lib_State_Machine.vi"("State(s) in (\"\")"=w350) -> ("States Out"=w349:string)  [unwired: 14 in]
      }
      frame "Library: Rename VIs" {
        # "Template Separator\n(You can make a copy of, or modify, this frame)"
        n128 = Unbundle By Name(w355) -> ("ProjectItem"=w356:refnum<class "ProjectItem.lvclass">)  [unwired: 2 out]
        n129 = call "Rename VIs.vi"("error in (no error)"=w352, "ProjectItem in"=w356) -> ("error out"=w351:errorcluster, "ProjectItem out"=w353:refnum<class "ProjectItem.lvclass">)  [unwired: 8 in]
        n130 = Bundle By Name(cluster=w355, "ProjectItem"=w353) -> (w354:T4)
        n131 = call <vilib>:"Add State(s) to Queue__JKI_lib_State_Machine.vi"("State(s) in (\"\")"=w358) -> ("States Out"=w357:string)  [unwired: 14 in]
      }
      frame "Library: Rename Controls" {
        # "Template Separator\n(You can make a copy of, or modify, this frame)"
        n132 = Unbundle By Name(w363) -> ("ProjectItem"=w364:refnum<class "ProjectItem.lvclass">)  [unwired: 2 out]
        n133 = call "Rename Typedefs.vi"("error in (no error)"=w360, "ProjectItem in"=w364) -> ("error out"=w359:errorcluster, "ProjectItem out"=w361:refnum<class "ProjectItem.lvclass">)  [unwired: 8 in]
        n134 = Bundle By Name(cluster=w363, "ProjectItem"=w361) -> (w362:T4)
        n135 = call <vilib>:"Add State(s) to Queue__JKI_lib_State_Machine.vi"("State(s) in (\"\")"=w366) -> ("States Out"=w365:string)  [unwired: 14 in]
      }
      frame "Library: Rename GObjects" {
        # "Template Separator\n(You can make a copy of, or modify, this frame)"
        n136 = Unbundle By Name(w371) -> ("ProjectItem"=w372:refnum<class "ProjectItem.lvclass">)  [unwired: 2 out]
        n137 = call "Rename GObjects.vi"("error in (no error)"=w368, "ProjectItem in"=w372) -> ("error out"=w367:errorcluster, "ProjectItem out"=w369:refnum<class "ProjectItem.lvclass">)  [unwired: 8 in]
        n138 = Bundle By Name(cluster=w371, "ProjectItem"=w369) -> (w370:T4)
        n139 = call <vilib>:"Add State(s) to Queue__JKI_lib_State_Machine.vi"("State(s) in (\"\")"=w374) -> ("States Out"=w373:string)  [unwired: 14 in]
      }
      frame "Library: Update Library Icons" {
        # "Template Separator\n(You can make a copy of, or modify, this frame)"
        n140 = Unbundle By Name(w379) -> ("ProjectItem"=w377:refnum<class "ProjectItem.lvclass">, "Instrument.Icon"=w376:refnum<class "Icon.lvclass">, "Instrument UI.Icon"=w375:refnum<class "Icon.lvclass">)
        n141 = call "Update Class Icon.vi"("error in (no error)"=w382, "UI Icon"=w375, "Icon"=w376, "Rename in"=w377) -> ("error out"=w381:errorcluster, "Rename out"=w378:refnum<class "ProjectItem.lvclass">)  [unwired: 6 in]
        n142 = Bundle By Name(cluster=w379, "ProjectItem"=w378) -> (w380:T4)
        n143 = call <vilib>:"Add State(s) to Queue__JKI_lib_State_Machine.vi"("State(s) in (\"\")"=w384) -> ("States Out"=w383:string)  [unwired: 14 in]
      }
      frame "Library: Update Library Wires" {
        # "Template Separator\n(You can make a copy of, or modify, this frame)"
        n144 = Unbundle By Name(w389) -> ("ProjectItem"=w387:refnum<class "ProjectItem.lvclass">, "Instrument.Color"=w386:u32, "Instrument UI.Color"=w385:u32)
        n145 = call "Update Class Wire Appearance.vi"("error in (no error)"=w392, "UI Color"=w385, "Color"=w386, "ProjectItem in"=w387) -> ("error out"=w391:errorcluster, "ProjectItem out"=w388:refnum<class "ProjectItem.lvclass">)  [unwired: 6 in]
        n146 = Bundle By Name(cluster=w389, "ProjectItem"=w388) -> (w390:T4)
        n147 = call <vilib>:"Add State(s) to Queue__JKI_lib_State_Machine.vi"("State(s) in (\"\")"=w394) -> ("States Out"=w393:string)  [unwired: 14 in]
      }
      frame "Library: Close References" {
        # "Template Separator\n(You can make a copy of, or modify, this frame)"
        n148 = Unbundle By Name(w398) -> ("ProjectItem"=w397:refnum<class "ProjectItem.lvclass">)
        n149 = call "Close.vi"("error in (no error)"=w396, "ProjectItem in"=w397) -> ("error out"=w395:errorcluster)  [unwired: 8 in, 1 out]
        n150 = call <vilib>:"Add State(s) to Queue__JKI_lib_State_Machine.vi"("State(s) in (\"\")"=w400) -> ("States Out"=w399:string)  [unwired: 14 in]
      }
    }
  }
